vi "_Read.vi"(8 "error in (no error)":errorcluster, 11 "Lockin SR830 in":refnum<class "Lockin SR830.lvclass">) -> (0 "error out":errorcluster, 2 "4 Data Points":dbl[](array[numeric]), 3 "Lockin SR830 out":refnum<class "Lockin SR830.lvclass">)   [LabVIEW 2009, in "Lockin SR830.lvclass"]
uses:
  Lockin SR830.lvclass
  <vilib>/regexp/Match Regular Expression.xnode
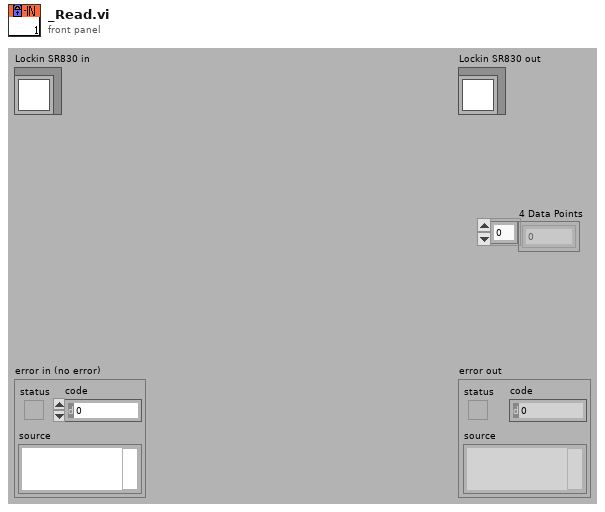
[diagram p1: front panel]
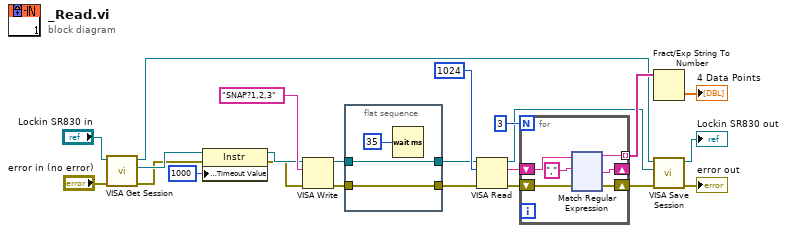
[diagram p0: block diagram]
diagram:
  n1 = call-dynamic "VISA Get Session.vi"("error in (no error)"="error in (no error)", "Instrument.lvclass in"="Lockin SR830 in") -> ("error out"=w3:errorcluster, "VISA Resource Name"=w4:refnum<visa-resource-name>, "Instrument.lvclass out"=w17:refnum<class "Lockin SR830.lvclass">)  [unwired: 7 out]
  n2 = property class="Instr"(reference=w4, error in=w3, "General Settings:Timeout Value"=u32 1000) -> (reference out=w2:refnum<visa-resource-name>, error out=w1:errorcluster)
  n3 = VISA Write(VISA resource name=w2, write buffer="SNAP?1,2,3", error in (no error)=w1) -> (VISA resource name out=w11:refnum<visa-resource-name>, error out=w9:errorcluster)  [unwired: 1 out]
  n4 = flat-sequence {
    tunnel: [w25] -> w10
    tunnel: w11 -> [w25]
    tunnel: [w24] -> w8
    tunnel: w9 -> [w24]
    frame #0 {
      n5 = Wait (ms)(milliseconds to wait=u32 35) -> ()  [unwired: 1 out]
    }
  }
  n6 = VISA Read(VISA resource name=w10, byte count=1024, error in (no error)=w8) -> (VISA resource name out=w7:refnum<visa-resource-name>, read buffer=w14:string, error out=w13:errorcluster)  [unwired: 1 out]
  n7 = for {
    N: 3 -> [_]
    tunnel: [w31] -> w19 mode=indexing
    shift-right: [w30] -> _
    shift-left: w14 -> [w29]
    shift-right: [w27] -> w6
    shift-left: w13 -> [w28]
    n8 = xnode "Match Regular Expression"("input string"=w29, "regular expression"=",", "error in"=w28) -> ("before match"=w31:string, "after match"=w30:string, "error out"=w27:errorcluster)  [unwired: 3 in, 2 out]
  }
  n9 = Fract/Exp String To Number(string=w19) -> (number=→"4 Data Points":dbl[])  [unwired: 3 in, 1 out]
  n10 = call-dynamic "VISA Save Session.vi"("error in (no error)"=w6, "VISA Resource Name"=w7, "Instrument.lvclass in"=w17) -> ("error out"=→"error out":errorcluster, "Instrument.lvclass out"=→"Lockin SR830 out":refnum<class "Lockin SR830.lvclass">)  [unwired: 7 out]
